vi "Timed Button Press.vi"(10 "Time Target (s)":dbl=1.0, 11 "Boolean 2":bool) -> (3 "Boolean":bool)   [LabVIEW 2016]
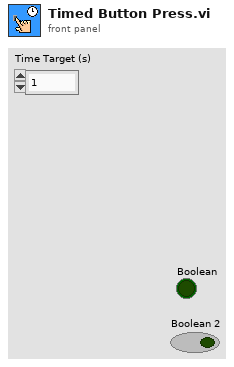
[diagram p1: front panel]
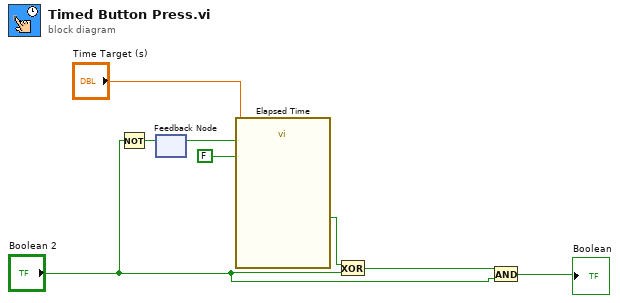
[diagram p0: block diagram]
diagram:
  n1 = Not(x="Boolean 2") -> (.not. x?=w5:bool)
  n2 = feedback #1() -> (w8:bool)  [unwired: 1 in]
  n3 = feedback-in #1(w5) -> ()
  n4 = call "Elapsed Time"("Time Target (s)"="Time Target (s)", "Reset"=w8, "Auto Reset"=FALSE) -> ("Time has Elapsed"=w7:bool)  [unwired: 9 in, 7 out]
  n5 = Exclusive Or(1:"Boolean 2", 2:w7) -> (0:w4:bool)
  n6 = And(x=w4, y="Boolean 2") -> (x .and. y?=→"Boolean":bool)
